vi "Pre Launch Init.vi"(11 "Sample Error Manager in":refnum<class "Sample Error Manager.lvclass">) -> (0 "error out":errorcluster, 3 "Sample Error Manager out":refnum<class "Sample Error Manager.lvclass">)   [LabVIEW 2024, in "Sample Error Manager.lvlib" / "Sample Error Manager.lvclass"]
doc: "<p>(<strong>Filename</strong>: <span class=\"dnl\">Actor Framework.lvlib:Actor.lvclass:Pre Launch Init.vi</span>)</p>\n<p>Defines behavior that occurs after the <a href=\"nihelplauncher://docs/csh?context=lvcore_lvcomm_af_launch_nested_actor\">Launch Nested Actor</a> method is invoked but before the actor's Actor Core method begins running.</p>\n<p>By default, this method does nothing. A descendant class may override it to define behavior.</p>"
uses:
  Sample Error Manager.lvclass
  Sample Error Manager.lvclass/Sample Error Manager.ctl
  src/Error Reporting Actor/Error Manager/Error Manager/Error Manager.lvclass
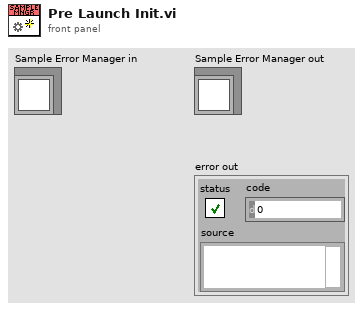
[diagram p1: front panel]
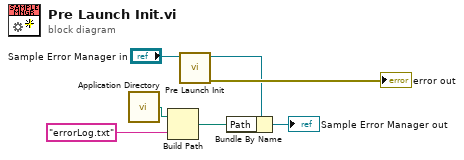
[diagram p0: block diagram]
diagram:
  n1 = call <vilib>:"Application Directory.vi"() -> ("Application Directory"=w5:path)
  n2 = Build Path(base path=w5, name or relative path="errorLog.txt") -> (appended path=w2:path)
  n3 = call-parent "Pre Launch Init.vi"("Actor in"="Sample Error Manager in") -> ("error out"=→"error out":errorcluster, "Actor out"=w3:refnum<class "Sample Error Manager.lvclass">)  [unwired: 9 in]
  n4 = Bundle By Name(cluster=w3, "Path"=w2) -> (→"Sample Error Manager out":refnum<class "Sample Error Manager.lvclass">)
